vi "Report Disconnect Error.vi"(8 "error in (no error)":errorcluster) -> (0 "error out":errorcluster)   [LabVIEW 2020, in "Communication VIs.lvlib" / "Local.lvlib"]
uses:
  <vilib>/Utility/error.llb/Error Cluster From Error Code.vi
  <vilib>/ErrorRing/Error Ring.xnode
  Local.lvlib
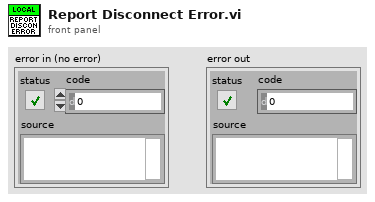
[diagram p1: front panel]
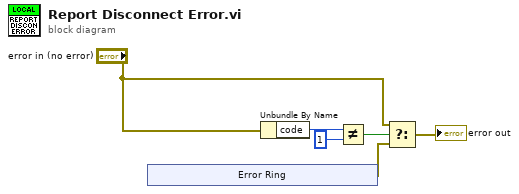
[diagram p0: block diagram]
diagram:
  n1 = xnode "Error Ring"() -> ("error out"=w5:errorcluster)
  n2 = Unbundle By Name("error in (no error)") -> ("code"=w2:i32)
  n3 = Not Equal?(x=w2, y=1) -> (x != y?=w1:bool)
  n4 = Select(t="error in (no error)", s=w1, f=w5) -> (s? t:f=→"error out":errorcluster)
